vi "Update Plots.vi"(8 "error in (no error)":errorcluster, 10 "File Path":path, 11 "Measure Controller in":refnum<class "Process Controller.lvclass">) -> (0 "error out":errorcluster, 3 "Measure Controller out":refnum<class "Process Controller.lvclass">)   [LabVIEW 2016, in "Process Controller.lvclass"]
uses:
  Process Controller.lvclass
  Process Controller.lvclass/Process Controller.ctl
  Plots/XY Plot Messages/File updated Msg/File updated Msg.lvclass/File updated Msg.ctl
  <vilib>/ActorFramework/Message Enqueuer/Message Enqueuer.lvclass/Message Enqueuer.ctl
  <vilib>/ActorFramework/Message Enqueuer/Enqueue.vi
  Plots/XY Plot Messages/File updated Msg/File updated Msg.lvclass
  D:/Program Files/National Instruments/LabVIEW 2016/vi.lib/ActorFramework/Message/Message.lvclass
  <vilib>/ActorFramework/Message Priority Queue/Priority Enqueue.vi
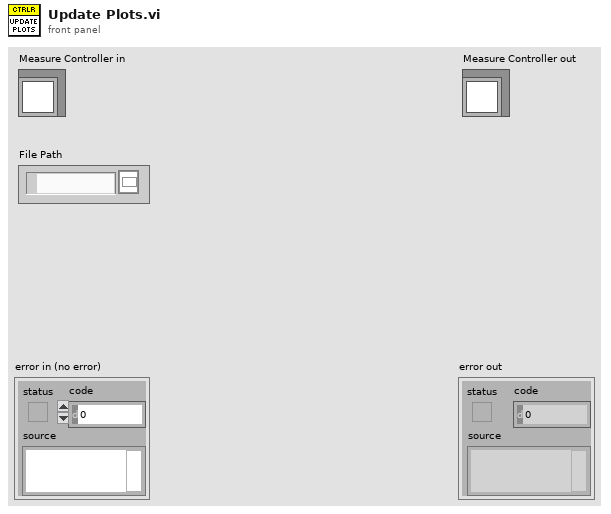
[diagram p1: front panel]
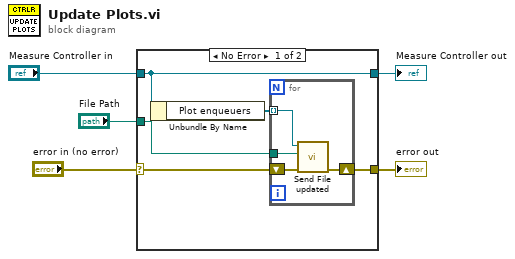
[diagram p0: block diagram]
diagram:
  n1 = case shown="No Error" "error in (no error)" {
    selector: "error in (no error)" -> [w7 w16]
    tunnel: [w6 w16] -> w4
    tunnel: [w10 w15] -> w2
    tunnel: "Measure Controller in" -> [w10 w15]
    tunnel: "File Path" -> [w8 _]
    frame No Error {
      n2 = Unbundle By Name(w10) -> ("Plot enqueuers"=w9:refnum<class "Message Enqueuer.lvclass">[])
      n3 = for {
        tunnel: w9 -> [w14] mode=indexing
        tunnel: w8 -> [w13]
        shift-right: [w11] -> w6
        shift-left: w7 -> [w12]
        n4 = call "Send File updated.vi"("error in (no error)"=w12, "File Path Control"=w13, "Message Enqueuer"=w14) -> ("error out"=w11:errorcluster)  [unwired: 7 in, 1 out]
      }
    }
    frame Error {
    }
  }
  "error out" <- w4
  "Measure Controller out" <- w2
